vi "TDMS Copy Group.vi"(6 "Group Name to Copy To":string, 7 "Group Name to Copy":string, 8 "error in (no error)":errorcluster, 10 "TDMS File to Copy To":refnum<k34>, 11 "TDMS File to Copy From":refnum<k34>) -> (0 "error out":errorcluster, 2 "TDMS File to Copy To out":refnum<k34>, 3 "TDMS File to Copy From out":refnum<k34>)   [LabVIEW 2020, in "Utilities.lvlib"]
doc: "Copies all group properties and all channels and their associated properties and channel data to another group. It is okay if the copy from and copy to group have the same name (a common use case) if the TDMS files are distinct."
uses:
  Utilities.lvlib
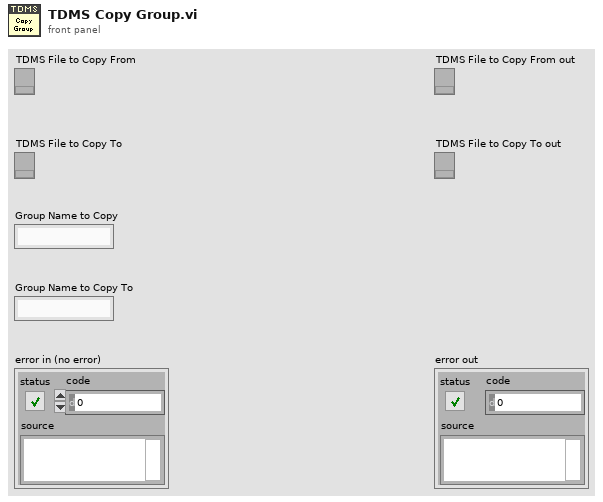
[diagram p1: front panel]
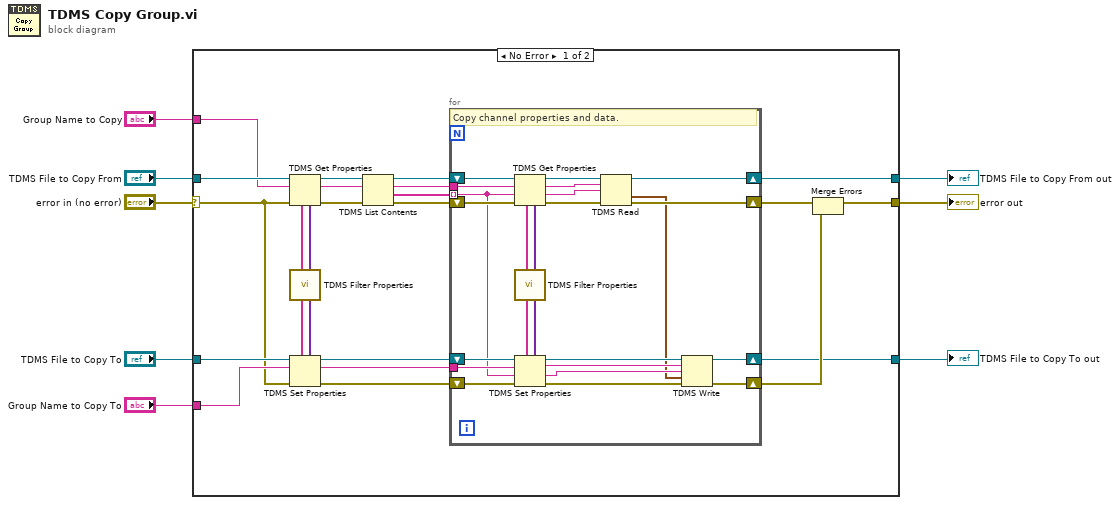
[diagram p0: block diagram]
diagram:
  n1 = case shown="No Error" "error in (no error)" {
    selector: "error in (no error)" -> [w9 w58]
    tunnel: "TDMS File to Copy From" -> [w22 w59]
    tunnel: "TDMS File to Copy To" -> [w21 w57]
    tunnel: "Group Name to Copy" -> [w20 _]
    tunnel: [w19 w59] -> w5
    tunnel: [w16 w57] -> w4
    tunnel: [w15 w58] -> w3
    tunnel: "Group Name to Copy To" -> [w14 _]
    frame No Error {
      n2 = TDMS Get Properties(8:w9, 10:w20, 11:w22) -> (0:w30:errorcluster, 2:w28:string, 3:w29:refnum<k34>, 4:w12:variant[], 6:w13:string[])  [unwired: 3 in, 1 out]
      n3 = call "TDMS Filter Properties.vi"("Property Values"=w12, "Property Names"=w13) -> ("Filtered Property Values"=w10:variant[], "Filtered Property Names"=w11:string[])  [unwired: 8 in]
      n4 = TDMS Set Properties(5:w10, 7:w11, 8:w9, 10:w14, 11:w21) -> (0:w26:errorcluster, 2:w23:string, 3:w27:refnum<k34>)  [unwired: 1 in, 1 out]
      n5 = TDMS List Contents(4:w30, 6:w28, 7:w29) -> (0:w24:errorcluster, 1:w31:string[], 2:w32:string, 3:w25:refnum<k34>)
      n6 = for {
        tunnel: w32 -> [w56]
        tunnel: w31 -> [w41] mode=indexing
        shift-right: [w44] -> w16
        shift-left: w27 -> [w55]
        shift-right: [w45] -> w17
        shift-left: w26 -> [w54]
        shift-right: [w38] -> w19
        shift-left: w25 -> [w53]
        shift-right: [w48] -> w18
        shift-left: w24 -> [w42]
        tunnel: w23 -> [w43]
        # "Copy channel properties and data."
        n7 = TDMS Get Properties(8:w42, 9:w41, 10:w56, 11:w53) -> (0:w51:errorcluster, 1:w49:string, 2:w50:string, 3:w52:refnum<k34>, 4:w36:variant[], 6:w37:string[])  [unwired: 2 in]
        n8 = call "TDMS Filter Properties.vi"("Property Values"=w36, "Property Names"=w37) -> ("Filtered Property Values"=w34:variant[], "Filtered Property Names"=w35:string[])  [unwired: 8 in]
        n9 = TDMS Set Properties(5:w34, 7:w35, 8:w54, 9:w41, 10:w43, 11:w55) -> (0:w46:errorcluster, 1:w40:string, 2:w39:string, 3:w47:refnum<k34>)
        n10 = TDMS Read(0:w52, 5:w50, 7:w49, 11:w51) -> (4:w38:refnum<k34>, 10:w33:waveform(dbl), 15:w48:errorcluster)  [unwired: 4 in, 3 out]
        n11 = TDMS Write(0:w47, 5:w39, 7:w40, 9:w33, 11:w46) -> (4:w44:refnum<k34>, 15:w45:errorcluster)  [unwired: 1 in, 2 out]
      }
      n12 = Merge Errors(w18, w17) -> (w15:errorcluster)
    }
    frame Error {
    }
  }
  "TDMS File to Copy From out" <- w5
  "TDMS File to Copy To out" <- w4
  "error out" <- w3
